vi "ExampleGratingsWavelength64.vi"() -> ()   [LabVIEW 2009]
panel:
  in  "Device":i32 min=0 max=0
  in  "Set Device":bool
  in  "Tab Control":enum32{"GRATINGS", "WAVELENGTH"}(tab)
  in  "Grating Offset":i32
  out "SetGratingOffset":string
  in  "Detector Offset":i32
  out "SetDetectorOffset":string
  out "WavelengthReset":string
  out "SetGrating":string
  in  "Grating":i32
  in  "Turret":i32
  out "SetTurret":string
  in  "SetGratingOffset":bool
  in  "SetDetectorOffset":bool
  in  "WavelengthReset":bool
  in  "SetGrating":bool
  in  "SetTurret":bool
  out "blaze":string
  out "Grating Offset":i32
  out "Detector Offset":i32
  out "offset":i32
  out "home":i32
  out "lines/mm":dbl format="%.2f"
  out "Grating":i32
  out "No Gratings":i32
  out "Turret":i32
  out "Is Grating ?":string
  out "GetGratingOffset":string
  out "GetDetectorOffset":string
  out "GetGratingInfo":string
  out "GetGrating":string
  out "GetNumberGratings":string
  out "GetTurret":string
  out "GratingIsPresent":string
  out "GotoZeroOrder":string
  out "SetWavelength":string
  in  "Wavelength":dbl format="%.2f"
  in  "GoToZeroOrder":bool
  out "Max Wavelength":dbl format="%.2f"
  out "Min Wavelength":dbl format="%.2f"
  out "Is Wavelength ?":string
  out "WavelengthIsPresent":string
  out "GetWavelengthLimits":string
  out "At Zero Order ?":string
  out "AtZeroOrder":string
  out "Wavelength":dbl format="%.2f"
  in  "SetWavelength 2":bool
  out "GetWavelength":string
  out "Initializing":bool
  in  "STOP if TRUE":bool
  out "Focal tilt":dbl format="%.2f"
  out "Angular deviation":dbl format="%.2f"
  out "Focal length":dbl format="%.2f"
  out "Serial Number":string
  out "No of devices":i32
  out "GetOpticalParameters":string
  out "GetSerialNumber":string
  out "GetNumberDevices":string
  out "Close":string
  out "Initialize":string
  # "INITIALIZATION"
  # "SDK RETURN VALUES"
  # "SHAMROCK PARAMETERS"
  # "ACTIONS"
  # "SDK RETURN VALUES"
  # "SHAMROCK PARAMETERS"
  # "ACTIONS"
  # "SDK RETURN VALUES"
  # "SHAMROCK PARAMETERS"
  # "ACTIONS"
  # "nm"
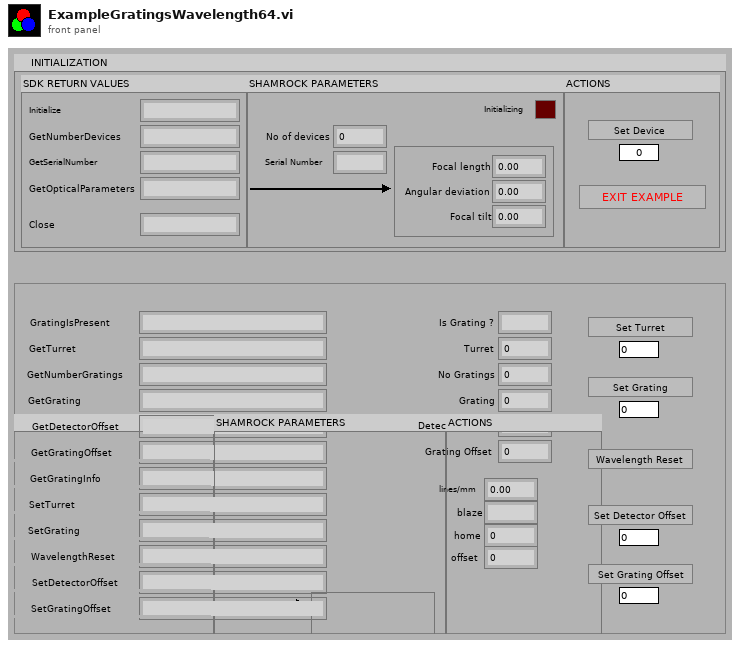
[diagram p1: front panel]
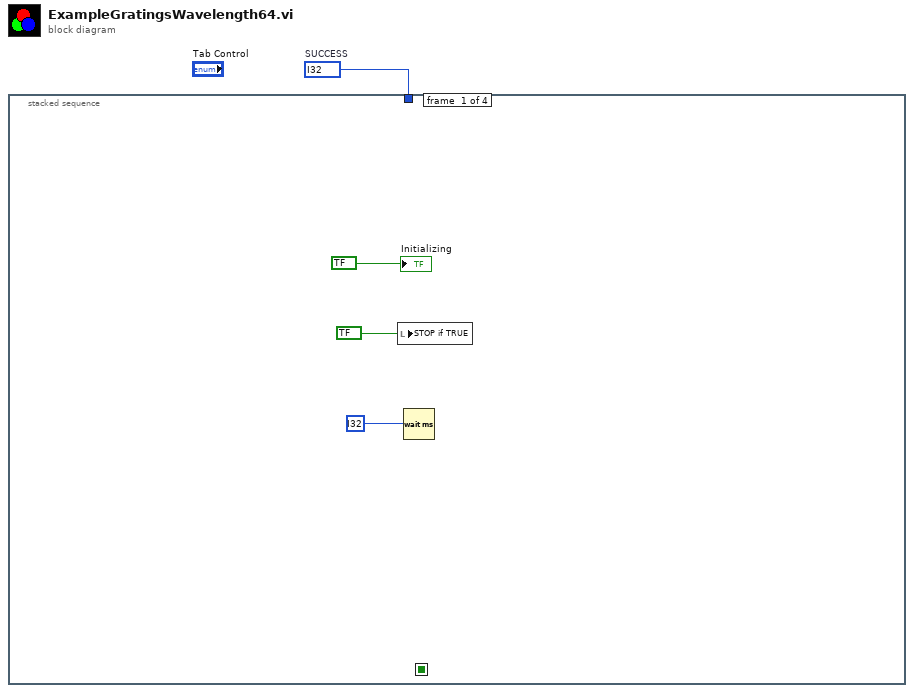
[diagram p0: block diagram]
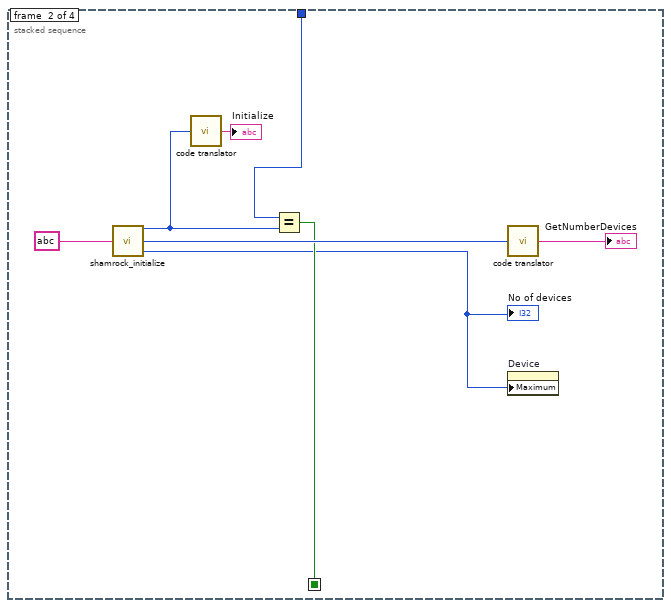
[diagram p2: hidden frame]
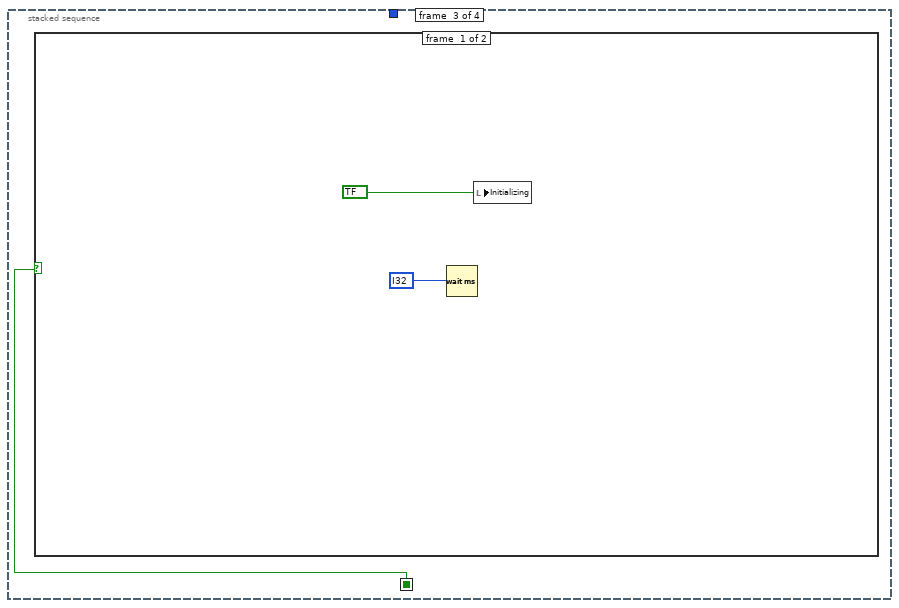
[diagram p3: hidden frame]
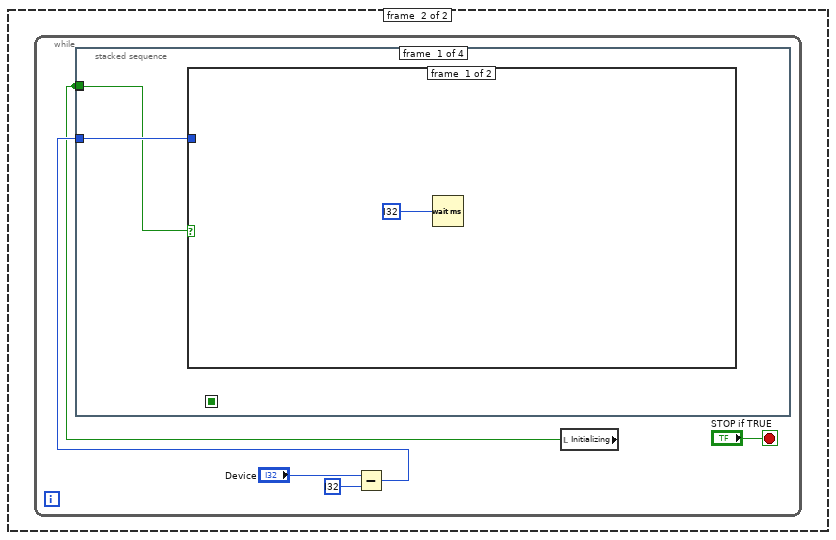
[diagram p4: hidden frame]
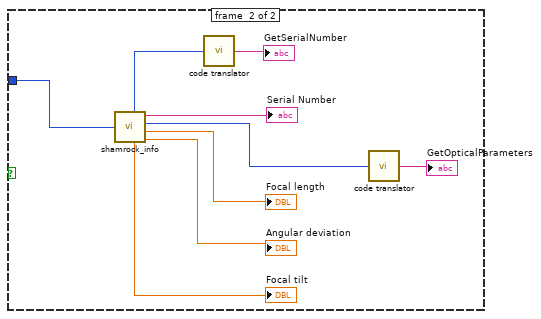
[diagram p5: hidden frame]
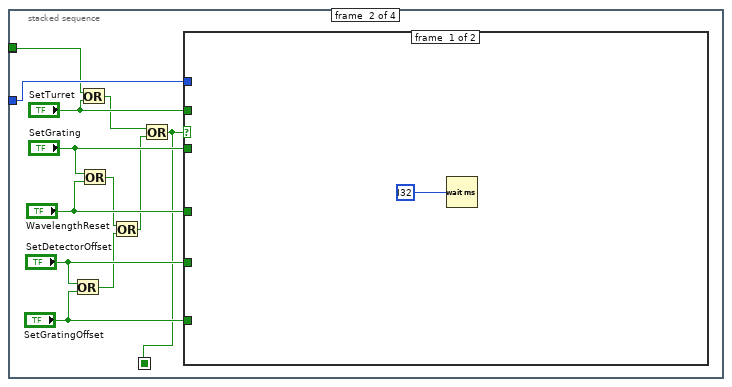
[diagram p6: hidden frame]
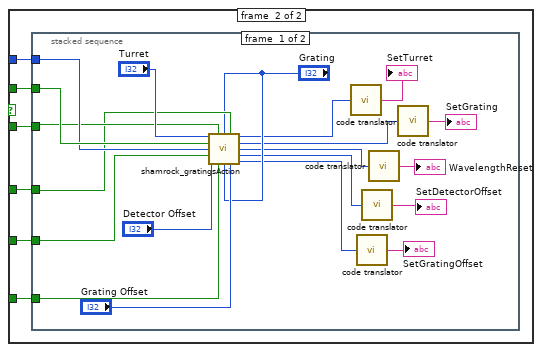
[diagram p7: hidden frame]
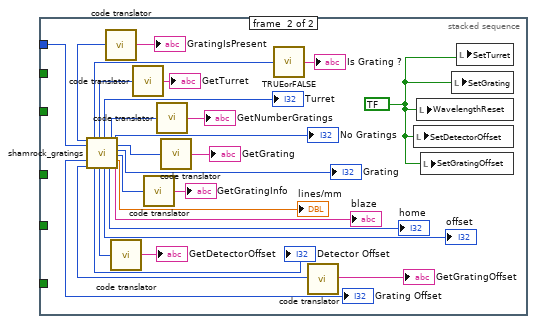
[diagram p8: hidden frame]
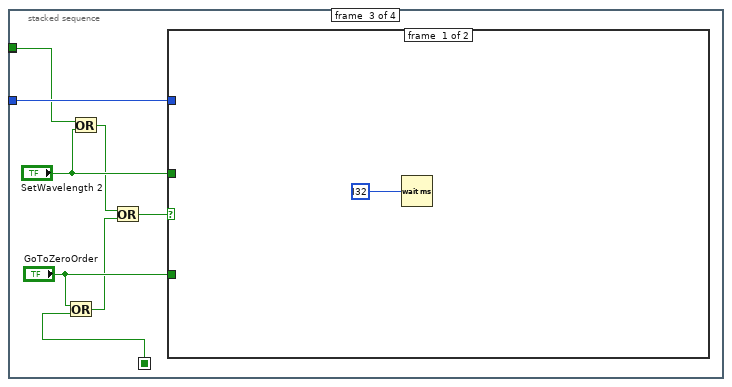
[diagram p9: hidden frame]
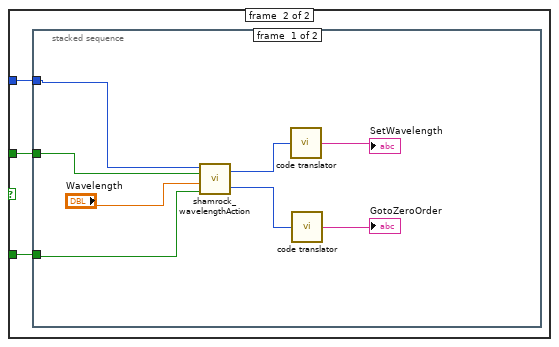
[diagram p10: hidden frame]
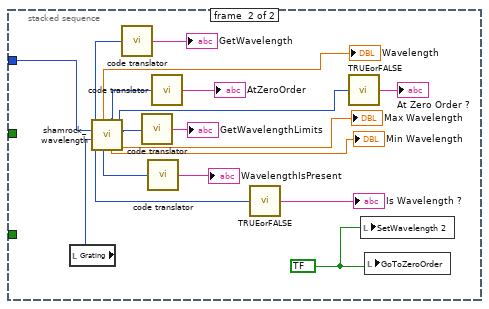
[diagram p11: hidden frame]
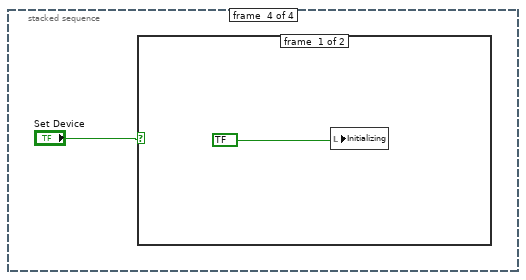
[diagram p12: hidden frame]
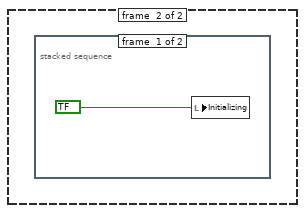
[diagram p13: hidden frame]
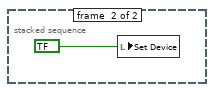
[diagram p14: hidden frame]
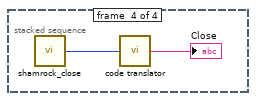
[diagram p15: hidden frame]
diagram:
  w1 = i32 ?  # SUCCESS
  n1 = stacked-sequence {
    seq-local: [_ w6 _ _] -> [_ _ w13 _]
    tunnel: w1 -> [_ w12 _ _]
    frame #0 {
      n2 = local write "STOP if TRUE"(bool ?) -> ()
      n3 = Wait (ms)(milliseconds to wait=i32 ?) -> ()  [unwired: 1 out]
      "Initializing" <- bool ?
    }
    frame #1 {
      n4 = call <userlib>:"shamrock_initialize.vi"("Initialization path"=string ?) -> ("Initialize"=w9:u32, "GetNumberDevices"=w8:u32, "No of devices"=w5:i32)
      "No of devices" <- w5
      n5 = call <userlib>:"code translator.vi"("Error code"=w9) -> ("Error description"=→"Initialize":string)
      n6 = Equal?(x=w12, y=w9) -> (x = y?=w6:bool)
      n7 = call <userlib>:"code translator.vi"("Error code"=w8) -> ("Error description"=→"GetNumberDevices":string)
      n8 = property on="Device" class="DigNum (strict)"("Maximum"=w5) -> ()  [unwired: 2 in, 2 out]
    }
    frame #2 {
      n9 = case shown="True" w13 {
        frame #0 {
          n10 = Wait (ms)(milliseconds to wait=i32 ?) -> ()  [unwired: 1 out]
          n11 = local write "Initializing"(bool ?) -> ()
        }
        frame #1 {
          n12 = while {
            stop <- "STOP if TRUE" stop-if-true
            n13 = Subtract(x="Device", y=i32 ?) -> (x-y=w19:i32)
            n14 = local read "Initializing"() -> (w16:bool)
            n15 = stacked-sequence {
              seq-local: [_ w33 _ _] -> [_ _ w105 _]
              tunnel: w19 -> [w22 w44 w106 _]
              tunnel: w16 -> [w21 w36 w102 _]
              tunnel: w16 -> [_ _ _ _]
              frame #0 {
                n16 = case shown="True" w21 {
                  tunnel: w22 -> [_ w24]
                  frame #0 {
                    n17 = Wait (ms)(milliseconds to wait=i32 ?) -> ()  [unwired: 1 out]
                  }
                  frame #1 {
                    n18 = call <userlib>:"shamrock_info.vi"("Device No"=w24) -> ("GetSerialNumber"=w28:u32, "Focal tilt"=→"Focal tilt":sgl, "Serial Number"=→"Serial Number":string, "GetOpticalParameters"=w26:u32, "Focal length"=→"Focal length":sgl, "Angular deviation"=→"Angular deviation":sgl)
                    n19 = call <userlib>:"code translator.vi"("Error code"=w28) -> ("Error description"=→"GetSerialNumber":string)
                    n20 = call <userlib>:"code translator.vi"("Error code"=w26) -> ("Error description"=→"GetOpticalParameters":string)
                  }
                }
              }
              frame #1 {
                n21 = Or(x="SetDetectorOffset", y="SetGratingOffset") -> (x .or. y?=w38:bool)
                n22 = Or(x=w36, y="SetTurret") -> (x .or. y?=w35:bool)
                n23 = Or(x="SetGrating", y="WavelengthReset") -> (x .or. y?=w39:bool)
                n24 = Or(x=w39, y=w38) -> (x .or. y?=w34:bool)
                n25 = Or(x=w35, y=w34) -> (x .or. y?=w33:bool)
                n26 = case shown="True" w33 {
                  tunnel: w44 -> [_ w51]
                  tunnel: "SetDetectorOffset" -> [_ w50]
                  tunnel: "SetGratingOffset" -> [_ w49]
                  tunnel: "SetGrating" -> [_ w48]
                  tunnel: "WavelengthReset" -> [_ w47]
                  tunnel: "SetTurret" -> [_ w46]
                  frame #0 {
                    n27 = Wait (ms)(milliseconds to wait=i32 ?) -> ()  [unwired: 1 out]
                  }
                  frame #1 {
                    n28 = stacked-sequence {
                      tunnel: w46 -> [w70 _]
                      tunnel: w51 -> [w69 w89]
                      tunnel: w48 -> [w64 _]
                      tunnel: w47 -> [w63 _]
                      tunnel: w50 -> [w68 _]
                      tunnel: w49 -> [w66 _]
                      frame #0 {
                        n29 = call <userlib>:"shamrock_gratingsAction.vi"("WavelengthReset"=w63, "Grating Offset"="Grating Offset", 7:"Grating"="Grating", 8:"Grating"="Grating", "SetGrating"=w64, "SetGratingOffset"=w66, "Turret"="Turret", "SetTurret"=w70, "Device No"=w69, "SetDetectorOffset"=w68, "Detector Offset"="Detector Offset") -> ("SetTurret"=w61:u32, "SetGrating"=w59:u32, "WavelengthReset"=w56:u32, "SetDetectorOffset"=w54:u32, "SetGratingOffset"=w53:u32)
                        n30 = call <userlib>:"code translator.vi"("Error code"=w61) -> ("Error description"=→"SetTurret":string)
                        n31 = call <userlib>:"code translator.vi"("Error code"=w53) -> ("Error description"=→"SetGratingOffset":string)
                        n32 = call <userlib>:"code translator.vi"("Error code"=w54) -> ("Error description"=→"SetDetectorOffset":string)
                        n33 = call <userlib>:"code translator.vi"("Error code"=w56) -> ("Error description"=→"WavelengthReset":string)
                        n34 = call <userlib>:"code translator.vi"("Error code"=w59) -> ("Error description"=→"SetGrating":string)
                      }
                      frame #1 {
                        w98 = bool ?
                        n35 = call <userlib>:"shamrock_gratings.vi"("Device No"=w89) -> ("No Gratings"=→"No Gratings":i32, "GetNumberGratings"=w83:u32, "Turret"=→"Turret":i32, "GetTurret"=w85:u32, "0:FALSE / 1:TRUE"=w73:i32, "GratingIsPresent"=w87:u32, "GetGrating"=w81:u32, "Grating"=→"Grating":i32, "GetGratingInfo"=w79:u32, "lines/mm"=→"lines/mm":dbl, "Grating Offset"=→"Grating Offset":i32, "blaze"=→"blaze":string, "home"=→"home":i32, "offset"=→"offset":i32, "GetDetectorOffset"=w77:u32, "Detector Offset"=→"Detector Offset":i32, "GetGratingOffset"=w75:u32)  [unwired: 2 in]
                        n36 = call <userlib>:"code translator.vi"("Error code"=w87) -> ("Error description"=→"GratingIsPresent":string)
                        n37 = call <userlib>:"code translator.vi"("Error code"=w77) -> ("Error description"=→"GetDetectorOffset":string)
                        n38 = call <userlib>:"code translator.vi"("Error code"=w85) -> ("Error description"=→"GetTurret":string)
                        n39 = call <userlib>:"code translator.vi"("Error code"=w79) -> ("Error description"=→"GetGratingInfo":string)
                        n40 = call <userlib>:"code translator.vi"("Error code"=w83) -> ("Error description"=→"GetNumberGratings":string)
                        n41 = call <userlib>:"code translator.vi"("Error code"=w81) -> ("Error description"=→"GetGrating":string)
                        n42 = call <userlib>:"TRUEorFALSE.vi"("bool number"=w73) -> ("String"=→"Is Grating ?":string)
                        n43 = call <userlib>:"code translator.vi"("Error code"=w75) -> ("Error description"=→"GetGratingOffset":string)
                        n44 = local write "SetDetectorOffset"(w98) -> ()
                        n45 = local write "WavelengthReset"(w98) -> ()
                        n46 = local write "SetGratingOffset"(w98) -> ()
                        n47 = local write "SetGrating"(w98) -> ()
                        n48 = local write "SetTurret"(w98) -> ()
                      }
                    }
                  }
                }
              }
              frame #2 {
                n49 = Or(x="GoToZeroOrder", y=w105) -> (x .or. y?=w100:bool)
                n50 = Or(x=w102, y="SetWavelength 2") -> (x .or. y?=w101:bool)
                n51 = Or(x=w101, y=w100) -> (x .or. y?=w99:bool)
                n52 = case shown="True" w99 {
                  tunnel: "SetWavelength 2" -> [_ w110]
                  tunnel: "GoToZeroOrder" -> [_ w109]
                  tunnel: w106 -> [_ w108]
                  frame #0 {
                    n53 = Wait (ms)(milliseconds to wait=i32 ?) -> ()  [unwired: 1 out]
                  }
                  frame #1 {
                    n54 = stacked-sequence {
                      tunnel: w110 -> [w116 _]
                      tunnel: w109 -> [w117 _]
                      tunnel: w108 -> [w115 w131]
                      frame #0 {
                        n55 = call <userlib>:"shamrock_wavelengthAction.vi"("GoToZeroOrder"=w117, "Wavelength"="Wavelength", "SetWavelength"=w116, "Device No"=w115) -> ("GotoZeroOrder"=w112:u32, "SetWavelength"=w114:u32)
                        n56 = call <userlib>:"code translator.vi"("Error code"=w114) -> ("Error description"=→"SetWavelength":string)
                        n57 = call <userlib>:"code translator.vi"("Error code"=w112) -> ("Error description"=→"GotoZeroOrder":string)
                      }
                      frame #1 {
                        w136 = bool ?
                        n58 = local read "Grating"() -> (w132:i32)
                        n59 = call <userlib>:"shamrock_wavelength.vi"("Grating No"=w132, "Device No"=w131) -> (0:"0:FALSE / 1:TRUE"=w120:i32, "WavelengthIsPresent"=w124:u32, "Min wl"=→"Min Wavelength":dbl, "Max wl"=→"Max Wavelength":dbl, "GetWavelengthLimits"=w126:u32, "GetWavelength"=w130:u32, "Wavelength"=→"Wavelength":dbl, "AtZeroOrder"=w128:u32, 10:"0:FALSE / 1:TRUE"=w122:i32)
                        n60 = call <userlib>:"code translator.vi"("Error code"=w130) -> ("Error description"=→"GetWavelength":string)
                        n61 = call <userlib>:"code translator.vi"("Error code"=w126) -> ("Error description"=→"GetWavelengthLimits":string)
                        n62 = call <userlib>:"code translator.vi"("Error code"=w124) -> ("Error description"=→"WavelengthIsPresent":string)
                        n63 = call <userlib>:"code translator.vi"("Error code"=w128) -> ("Error description"=→"AtZeroOrder":string)
                        n64 = call <userlib>:"TRUEorFALSE.vi"("bool number"=w120) -> ("String"=→"Is Wavelength ?":string)
                        n65 = call <userlib>:"TRUEorFALSE.vi"("bool number"=w122) -> ("String"=→"At Zero Order ?":string)
                        n66 = local write "SetWavelength 2"(w136) -> ()
                        n67 = local write "GoToZeroOrder"(w136) -> ()
                      }
                    }
                  }
                }
              }
              frame #3 {
                n68 = case shown="True" "Set Device" {
                  frame #0 {
                    n69 = local write "Initializing"(bool ?) -> ()
                  }
                  frame #1 {
                    n70 = stacked-sequence {
                      frame #0 {
                        n71 = local write "Initializing"(bool ?) -> ()
                      }
                      frame #1 {
                        n72 = local write "Set Device"(bool ?) -> ()
                      }
                    }
                  }
                }
              }
            }
          }
        }
      }
    }
    frame #3 {
      n73 = call <userlib>:"shamrock_close.vi"() -> ("Close"=w142:u32)
      n74 = call <userlib>:"code translator.vi"("Error code"=w142) -> ("Error description"=→"Close":string)
    }
  }
